vi "Convert Modular DT Globals to Full System Format.vi"(9 "DT in":dbl[][](array[numeric]), 10 "DT FREQ in":dbl[][](array[numeric])) -> (1 "DT out":dbl[][](array[numeric]), 2 "DT FREQ out":dbl[][](array[numeric]))   [LabVIEW 2011]
uses:
  WebEngine/LIB/CAL/DT vs FREQ Global Data Index.ctl
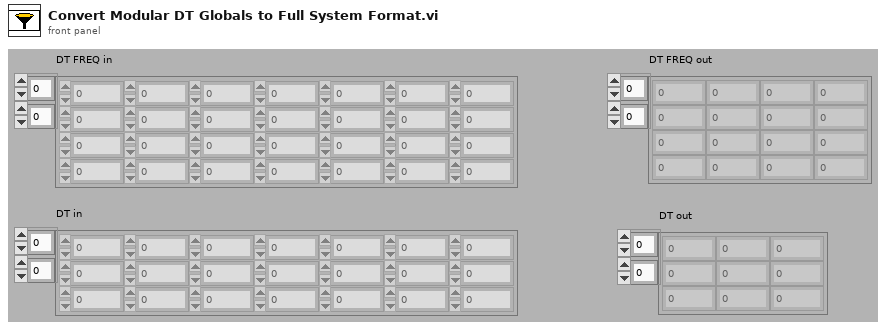
[diagram p1: front panel]
types:
  T1 = typedef "DT vs FREQ Global Data Index.ctl" = enum16{"Frequency, MHz", "Detector Voltage, DdB/DV", "Port, DdB", "VASegment Index", "FE Port 1 Loss, dB", "FE Port 2 Loss, dB"}
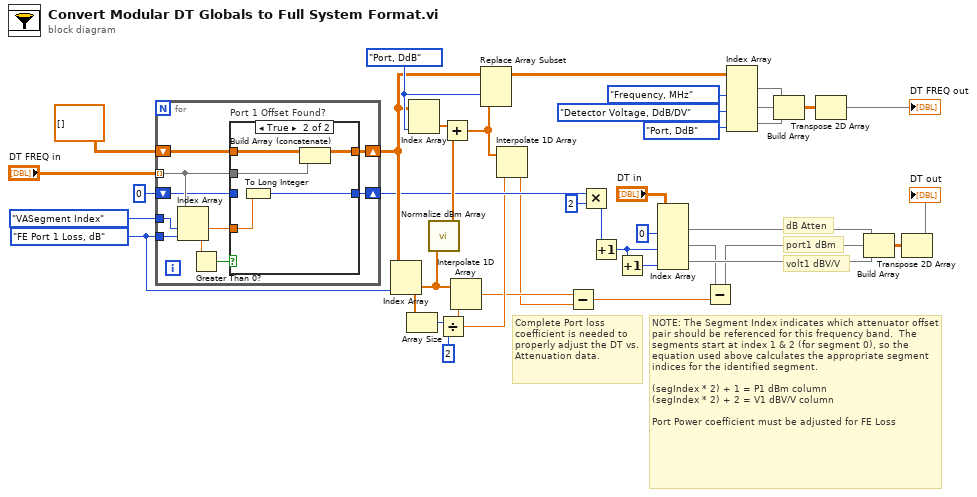
[diagram p0: block diagram]
diagram:
  w18 = DT_vs_FREQ_Global_Data_Index."Port, DdB" ("DT vs FREQ Global Data Index")
  w27 = DT_vs_FREQ_Global_Data_Index."FE Port 1 Loss, dB" ("DT vs FREQ Global Data Index")
  # "Complete Port loss coefficient is needed to properly adjust the DT vs. Attenuation data."
  # "volt1 dBV/V"
  # "port1 dBm"
  # "dB Atten"
  # "NOTE: The Segment Index indicates which attenuator offset pair should be referenced for this frequency band.  The segments start at index 1 & 2 (for segment 0), so the equation used above calculates the appropriate segment indices for the identified segment.\n\n(segIndex * 2) + 1 = P1 dBm column\n(segIndex * 2) + 2 = V1 dBV/V column\n\nPort Power coefficient must be adjusted for FE Loss"
  n1 = for {
    tunnel: "DT FREQ in" -> [w47] mode=indexing
    tunnel: w27 -> [w49]
    shift-right: [w40] -> w17
    shift-left: dbl[][] [] -> [w48]
    tunnel: DT_vs_FREQ_Global_Data_Index."VASegment Index" ("DT vs FREQ Global Data Index") -> [w44]
    shift-right: [w41] -> w7
    shift-left: 0 -> [w42]
    n2 = Index Array(array=w47, index #1=w44, index #2=w49) -> (element #1=w43:dbl, element #2=w45:dbl)
    n3 = Greater Than 0?(x=w45) -> (x > 0?=w46:bool)
    n4 = case "Port 1 Offset Found?" shown="True" w46 {
      tunnel: w48 -> [w50 w56]
      tunnel: w47 -> [_ w52]
      tunnel: w43 -> [_ w55]
      tunnel: w42 -> [w51 _]
      tunnel: [w51 w54] -> w41
      tunnel: [w50 w53] -> w40
      frame False {
      }
      frame True {
        n5 = To Long Integer(number=w55) -> (32bit integer=w54:i32)
        n6 = Build Array (concatenate)(w56, w52) -> (w53:dbl[][])
      }
    }
  }
  n7 = Index Array(array=w17, index (col)=w27) -> (element=w20:dbl[])  [unwired: 1 in]
  n8 = Array Size(array=w20) -> (size(s)=w26:i32)
  n9 = Index Array(array=w17, index (col)=w18) -> (element=w3:dbl[])  [unwired: 1 in]
  n10 = call "Normalize dBm Array.vi"("Input Array, dBm"=w20) -> ("Normalized Array, delta dB"=w19:dbl[])  [unwired: 4 in]
  n11 = Divide(x=w26, y=2) -> (x/y=w6:dbl)
  n12 = Add(x=w3, y=w19) -> (x+y=w2:dbl[])
  n13 = Interpolate 1D Array(1:w6, 2:w20) -> (0:w4:dbl)
  n14 = Replace Array Subset(array=w17, new element=w2, index (col)=w18) -> (w9:dbl[][])  [unwired: 1 in]
  n15 = Interpolate 1D Array(1:w6, 2:w2) -> (0:w1:dbl)
  n16 = Subtract(x=w4, y=w1) -> (x-y=w5:dbl)
  n17 = Multiply(x=w7, y=2) -> (x*y=w35:i32)
  n18 = Increment(x=w35) -> (x+1=w30:i32)
  n19 = Increment(x=w30) -> (x+1=w31:i32)
  n20 = Index Array(array="DT in", index (col) #1=0 ("disabled index (col)"), index (col) #2=w30, index (col) #3=w31) -> (element #1=w23:dbl[], element #2=w22:dbl[], element #3=w24:dbl[])  [unwired: 3 in]
  n21 = Subtract(x=w22, y=w5) -> (x-y=w21:dbl[])
  n22 = Index Array(array=w9, index (col) #1=DT_vs_FREQ_Global_Data_Index."Frequency, MHz" ("DT vs FREQ Global Data Index"), index (col) #2=DT_vs_FREQ_Global_Data_Index."Detector Voltage, DdB/DV" ("DT vs FREQ Global Data Index"), index (col) #3=DT_vs_FREQ_Global_Data_Index."Port, DdB" ("DT vs FREQ Global Data Index")) -> (element #1=w13:dbl[], element #2=w11:dbl[], element #3=w12:dbl[])  [unwired: 3 in]
  n23 = Build Array(w13, w11, w12) -> (w10:dbl[][])
  n24 = Transpose 2D Array(2D array=w10) -> (transposed array=→"DT FREQ out":dbl[][])
  n25 = Build Array(w23, w21, w24) -> (w29:dbl[][])
  n26 = Transpose 2D Array(2D array=w29) -> (transposed array=→"DT out":dbl[][])
